vi "AFG3022B_Init.vi"(0 "object in":refnum<class "AFG3022B.lvclass">, 2 "VISA resource name":refnum<visa-resource-name>, 5 "error in (no error)":errorcluster) -> (14 "object out":refnum<class "AFG3022B.lvclass">, 19 "error out":errorcluster)   [LabVIEW 2019, in "AFG3022B.lvclass"]
uses:
  AFG3022B.lvclass
  AFG3022B.lvclass/AFG3022B.ctl
  Tektronix AFG 3000 Series/Tektronix AFG 3000 Series.lvlib
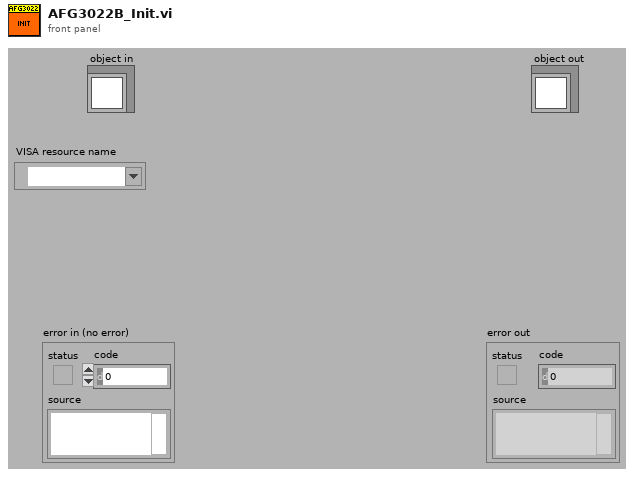
[diagram p1: front panel]
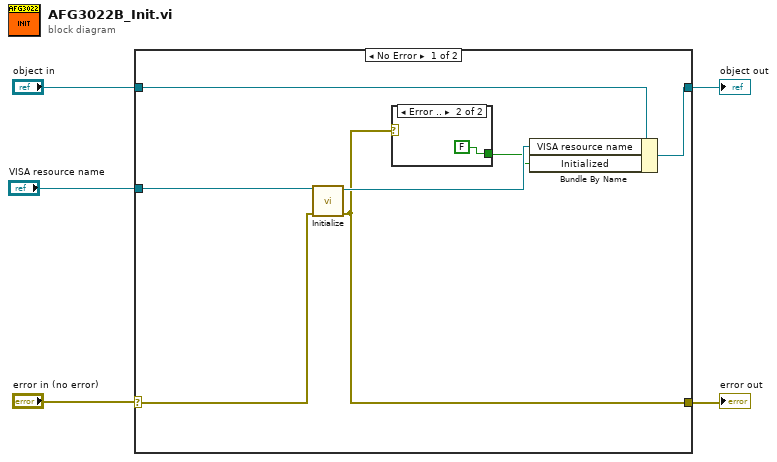
[diagram p0: block diagram]
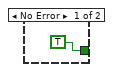
[diagram p2: hidden frame]
diagram:
  n1 = case shown="No Error" "error in (no error)" {
    selector: "error in (no error)" -> [w9 w15]
    tunnel: "object in" -> [w12 w16]
    tunnel: [w11 w16] -> w4
    tunnel: [w7 w15] -> w2
    tunnel: "VISA resource name" -> [w10 _]
    frame No Error {
      n2 = call "Initialize.vi"("error in (no error)"=w9, "VISA resource name"=w10) -> ("error out"=w7:errorcluster, "VISA resource name out"=w8:refnum<visa-resource-name>)  [unwired: 8 in]
      n3 = case shown="Error .." w7 {
        tunnel: [TRUE FALSE] -> w6
        frame No Error {
        }
        frame Error {
        }
      }
      n4 = Bundle By Name(cluster=w12, "VISA resource name"=w8, "Initialized"=w6) -> (w11:refnum<class "AFG3022B.lvclass">)
    }
    frame Error {
    }
  }
  "object out" <- w4
  "error out" <- w2
